vi "Create Pattern Script - Write Frame.vi"(8 "error in (no error)":errorcluster, 10 "FRM Data":T1 {"Addr" format="%x"; "Data" format="%x"}, 11 "SPI 3W Pattern Creator in":refnum<class "SPI 3W Pattern Creator.lvclass">) -> (0 "error out":errorcluster, 2 "String":string, 3 "SPI 3W Pattern Creator out":refnum<class "SPI 3W Pattern Creator.lvclass">)   [LabVIEW 2018, in "SPI 3W Pattern Creator.lvlib" / "SPI 3W Pattern Creator.lvclass"]
uses:
  SPI 3W Pattern Creator.lvclass
  C:/P4 Workspace/PC Client/Solutions/5g_eap/trunk/1.0/HiSi5GmmWave/Pattern_Gen_Tool/Interfaces/Protocol Interface.lvlibp/Interfaces/Protocol Interface/Protocol Interface.lvclass
  Ctls/Frame Data - SPI_3W.ctl
  Ctls/RW Options.ctl
  Protocols/SPI Root Pattern Creator.lvlibp/Plugins/SouceCode/SPI_Pattern Creator/SPI Root/Special Frame Type.ctl
  Protocols/SPI Root Pattern Creator.lvlibp/Plugins/SouceCode/SPI_Pattern Creator/SPI Root/Data Type.ctl
  Interfaces/Protocol Interface.lvlibp/Interfaces/Protocol Interface/Read Period(ms).vi
  Protocols/SPI Root Pattern Creator.lvlibp/Plugins/SouceCode/SPI_Pattern Creator/SPI Root/SPI Root Pattern Creator.lvclass
  C:/P4 Workspace/PC Client/Solutions/5g_eap/trunk/1.0/HiSi5GmmWave/Pattern_Gen_Tool/Plugins/Protocols/SPI Root Pattern Creator.lvlibp/Plugins/SouceCode/SPI_Pattern Creator/SPI Root/SPI Root Pattern Creator.lvclass
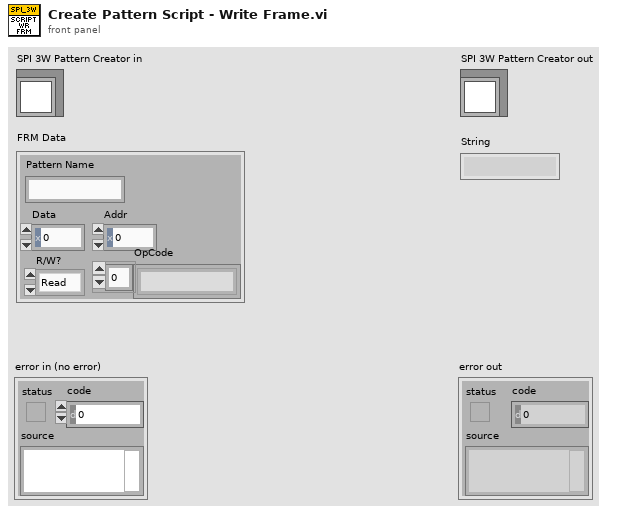
[diagram p1: front panel]
types:
  T1 = typedef "Frame Data - SPI_3W.ctl" = cluster{"Pattern Name":string, "Data":u16, "Addr":u16, "OpCode":string[], "R/W?":T2}
  T2 = typedef "RW Options.ctl" = enum16{"Read", "Write", "R/W"}
  T3 = typedef "SPI Root Pattern Creator.lvlibp/SPI Root Pattern Creator.lvclass/Data Type.ctl" = enum16{"Drive", "Compare", "Read"}
  T4 = typedef "SPI Root Pattern Creator.lvlibp/SPI Root Pattern Creator.lvclass/Special Frame Type.ctl" = enum16{"SPI 4W FRM Start", "SPI 4W Wait", "SPI 4W FRM End", "SPI 4W Write Cmd", "SPI Rd Collect Cmd", "SPI Rd Value Cmd", "SPI 3W FRM Start", "SPI 3W Write Cmd", "SPI 3W FRM End", "SPI 3W Wait", "SPI 3W Rd Cmd"}
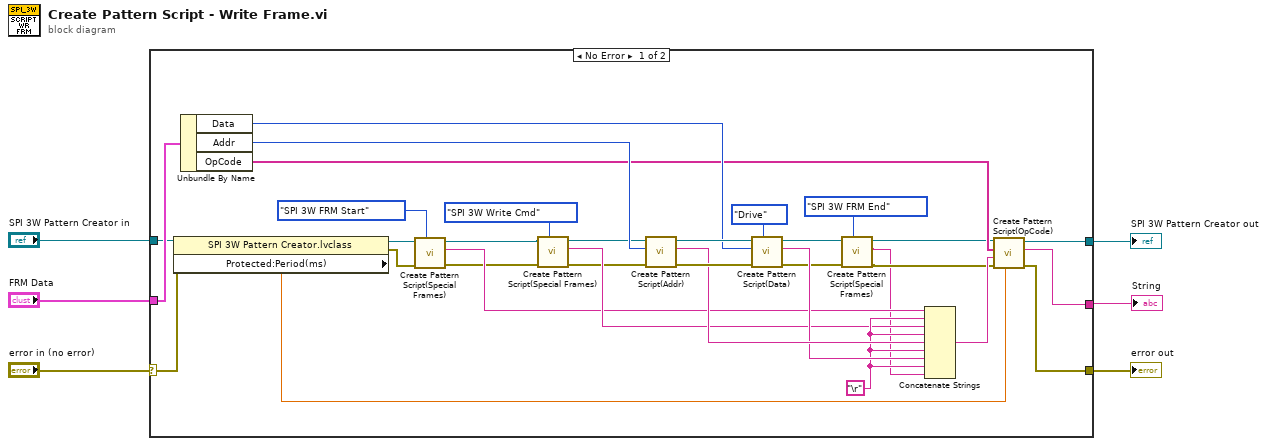
[diagram p0: block diagram]
diagram:
  n1 = case shown="No Error" "error in (no error)" {
    selector: "error in (no error)" -> [w24 w40]
    tunnel: "FRM Data" -> [w39 _]
    tunnel: "SPI 3W Pattern Creator in" -> [w31 w41]
    tunnel: [w29 w41] -> w3
    tunnel: [w28 _] -> w2
    tunnel: [w27 w40] -> w1
    frame No Error {
      w32 = "\r"
      n2 = property class="SPI 3W Pattern Creator.lvclass"(reference=w31, error in=w24) -> (reference out=w23:refnum<class "SPI 3W Pattern Creator.lvclass">, error out=w22:errorcluster, "Protected:Period(ms)"=w26:dbl)
      n3 = Unbundle By Name(w39) -> ("Data"=w35:u16, "Addr"=w36:u16, "OpCode"=w30:string[])
      n4 = call "Create Pattern Script(Special Frames).vi"("Special Frame Type"=Special_Frame_Type."SPI 3W FRM Start", "error in (no error)"=w22, "SPI Root Pattern Creator in"=w23) -> ("error out"=w17:errorcluster, "String out"=w18:string, "SPI Root Pattern Creator out"=w21:refnum<class "SPI 3W Pattern Creator.lvclass">)  [unwired: 6 in]
      n5 = call "Create Pattern Script(Special Frames).vi"("Special Frame Type"=Special_Frame_Type."SPI 3W Write Cmd", "error in (no error)"=w17, "SPI Root Pattern Creator in"=w21) -> ("error out"=w14:errorcluster, "String out"=w19:string, "SPI Root Pattern Creator out"=w20:refnum<class "SPI 3W Pattern Creator.lvclass">)  [unwired: 6 in]
      n6 = call-dynamic "Create Pattern Script(Addr).vi"("error in (no error)"=w14, "Addr"=w36, "SPI 3W Pattern Creator in"=w20) -> ("error out"=w38:errorcluster, "String"=w34:string, "SPI 3W Pattern Creator out"=w37:refnum<class "SPI 3W Pattern Creator.lvclass">)  [unwired: 6 in]
      n7 = call-dynamic "Create Pattern Script(Data).vi"("Data Type"=Data_Type."Drive", "error in (no error)"=w38, "Data"=w35, "SPI 3W Pattern Creator in"=w37) -> ("error out"=w11:errorcluster, "String"=w33:string, "SPI 3W Pattern Creator out"=w12:refnum<class "SPI 3W Pattern Creator.lvclass">)  [unwired: 5 in]
      n8 = call "Create Pattern Script(Special Frames).vi"("Special Frame Type"=Special_Frame_Type."SPI 3W FRM End", "error in (no error)"=w11, "SPI Root Pattern Creator in"=w12) -> ("error out"=w10:errorcluster, "String out"=w9:string, "SPI Root Pattern Creator out"=w8:refnum<class "SPI 3W Pattern Creator.lvclass">)  [unwired: 6 in]
      n9 = Concatenate Strings(w18, w32, w19, w32, w34, w32, w33, w32, w9) -> (w25:string)
      n10 = call "Create Pattern Script(OpCode).vi"("Period(ms)"=w26, "error in (no error)"=w10, "String in"=w25, "OpCode"=w30, "SPI 3W Pattern Creator in"=w8) -> ("error out"=w27:errorcluster, "String out"=w28:string, "SPI 3W Pattern Creator out"=w29:refnum<class "SPI 3W Pattern Creator.lvclass">)  [unwired: 4 in]
    }
    frame Error {
    }
  }
  "error out" <- w1
  "SPI 3W Pattern Creator out" <- w3
  "String" <- w2
